vi "Untitled 1.vi"() -> ()   [LabVIEW 2021]
panel:
  in  "Phase":dbl
  in  "Frequency":dbl=10.1
  out "Waveform Graph":dynamicdata(graph)
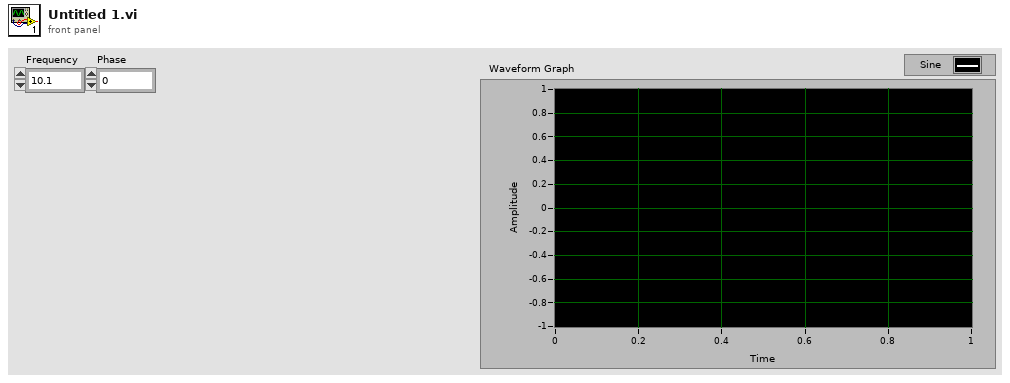
[diagram p1: front panel]
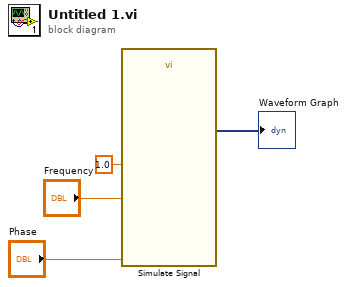
[diagram p0: block diagram]
diagram:
  n1 = call "Simulate Signal"("Frequency"="Frequency", "Amplitude"=1.0, "Phase"="Phase") -> ("Sine"=→"Waveform Graph":dynamicdata)  [unwired: 11 in, 1 out]
